vi "Launch XY Config Dialog.vi"(8 "error in (no error)":errorcluster, 11 "Waveform Graph Data in":T1={"Custom Data"=variant, "EventRegs"={"SystemChange"=refnum, "WorkspaceState"=refnum, "Graph"=refnum, "Wks&Dialog&Periodic"=refnum}, "References"={"X.Scale.Auto"=refnum, "Y.Scale.Auto"=refnum, "X.Scale.Once"=refnum, "Y.Scale.Once"=refnum, "LegendVis"=refnum, "Graph"=refnum}, "Persistent Data"={"Label"="", "Graph Props"={"Plots"=[], "Legend:Number of Rows"=0, "Scale Properties"={"X.Auto"=FALSE, "X.Min"=0.0, "X.Max"=0.0, "X.IgnoreTS"=FALSE, "X.Precision"=0, "X.Label:"="", "X.LabelVis"=FALSE, "X.DefLabel"=FALSE, "Y.Auto"=FALSE, "Y.Min"=0.0, "Y.Max"=0.0, "Y.Format"=0, "Y.Precision:"=0, "Y.Label:"="", "Y.LabelVis"=FALSE, "Y.DefLabel"=FALSE, "X.Format"=0}, "Legend:Visible"=TRUE, "BgColor"=0, "Last Plot Width"=0, "Resize"=FALSE}, "UDP Data"={"Decimation"=0, "UDP Buffer Size"=0, "History Length"=0.0, "Update Rate"=enum."15 Hz", "Channel Paths"=[], "Channel Names"=[]}}, "System"={"To Workspace"=refnum, "From Workspace"=refnum, "NIVS helper"=refnum, "Gtwy"="", "Root"=refnum, "Workspace"=refnum, "SystemStateRefs"={"CustDatRef"=refnum, "EvtRef"=refnum}, "Connected?"=FALSE, "FromDialog"=refnum, "ErrFlag"=FALSE, "New"=FALSE, "ErrState"="", "Save"=FALSE, "Hold"=FALSE, "Periodic"=refnum, "ToDialog"=refnum, "DialogEventReg"=refnum, "UseSavedWidth"=FALSE, "TreeBrowserEventReg"=refnum, "UDPChannelStreamSession"=refnum, "Valid Channels?"=FALSE, "Update Graph"=refnum, "UDP Queue"=refnum, "Graph Update Queue"=refnum}, "GraphData"=[], "UDP Stream Active?"=FALSE} {"Persistent Data"."Graph Props"."Scale Properties"."X.Format" items=["Decimal", "Scientific", "Engineering", "Binary", "Octal", "Hexadecimal", "Relative Time", "Time and Date", "SI", "Automatic"]; "Persistent Data"."Graph Props"."Scale Properties"."Y.Precision:" items=["0", "1", "2", "3", "4", "5", "6", "7"]; "Persistent Data"."Graph Props"."Scale Properties"."Y.Format" items=["Decimal", "Scientific", "Engineering", "Binary", "Octal", "Hexadecimal", "Relative Time", "Time and Date", "SI", "Automatic"]; "Persistent Data"."Graph Props"."Scale Properties"."X.Precision" items=["0", "1", "2", "3", "4", "5", "6", "7"]}) -> (0 "error out":errorcluster)   [LabVIEW 2013, in "Workspace MultiY Graph.lvlib"]
uses:
  Workspace MultiY Graph.lvlib
  XY Top level workspace graph data.ctl
  <vilib>/NI Veristand/Execution/Workspace/SystemStateRegEventRef.ctl
  <vilib>/NI Veristand/Display Template Support/Display Template Support.llb/enum_Display Template Handler Minimal To Widget Msg.ctl
  XY Dialog Msg to Control.ctl
  XY Dialog Msg Type.ctl
  XY Persistent Data.ctl
  XY Graph Properties.ctl
  XY Plot Properties.ctl
  XY Scale Properties.ctl
  XY Scale Precision.ctl
  XY Scale Format.ctl
  UDP Data.ctl
  Update Rate.ctl
  XY References.ctl
  <vilib>/NI Veristand/Display Template Support/Display Template Support.llb/enum_Display Template Handler Minimal To Workspace.ctl
  NationalInstruments.VeriStand.SystemStorage
  <vilib>/NI Veristand/Execution/Workspace/WorkspaceAPI.ctl
  NationalInstruments.VeriStand.ClientAPI
  <vilib>/NI Veristand/Execution/Workspace/SystemStateEventRef.ctl
  XY Control Msg to Dialog.ctl
  <vilib>/NI Veristand/UI Controls/Tree and Alias Browser/Net Event Data Ref.ctl
  <vilib>/NI Veristand/UI Controls/Tree and Alias Browser/Net Event Data.ctl
  <vilib>/NI Veristand/UI Controls/Tree and Alias Browser/Net Event.ctl
  <vilib>/NI Veristand/Execution/Workspace/UDPChannelStreamSession.ctl
  UDP Queue Data.ctl
  UDP Action State.ctl
  Graph Update Queue Data.ctl
  Graph Update Action State.ctl
  Dlg Symbol.ctl
  Alert Dialogs.lvlib
  <vilib>/NI Veristand/Execution/Workspace/NI_VS Workspace ExecutionAPI.lvlib
  <vilib>/NI Veristand/UI Controls/Tree and Alias Browser/NI_VS UI Tree Alias Browser.lvlib
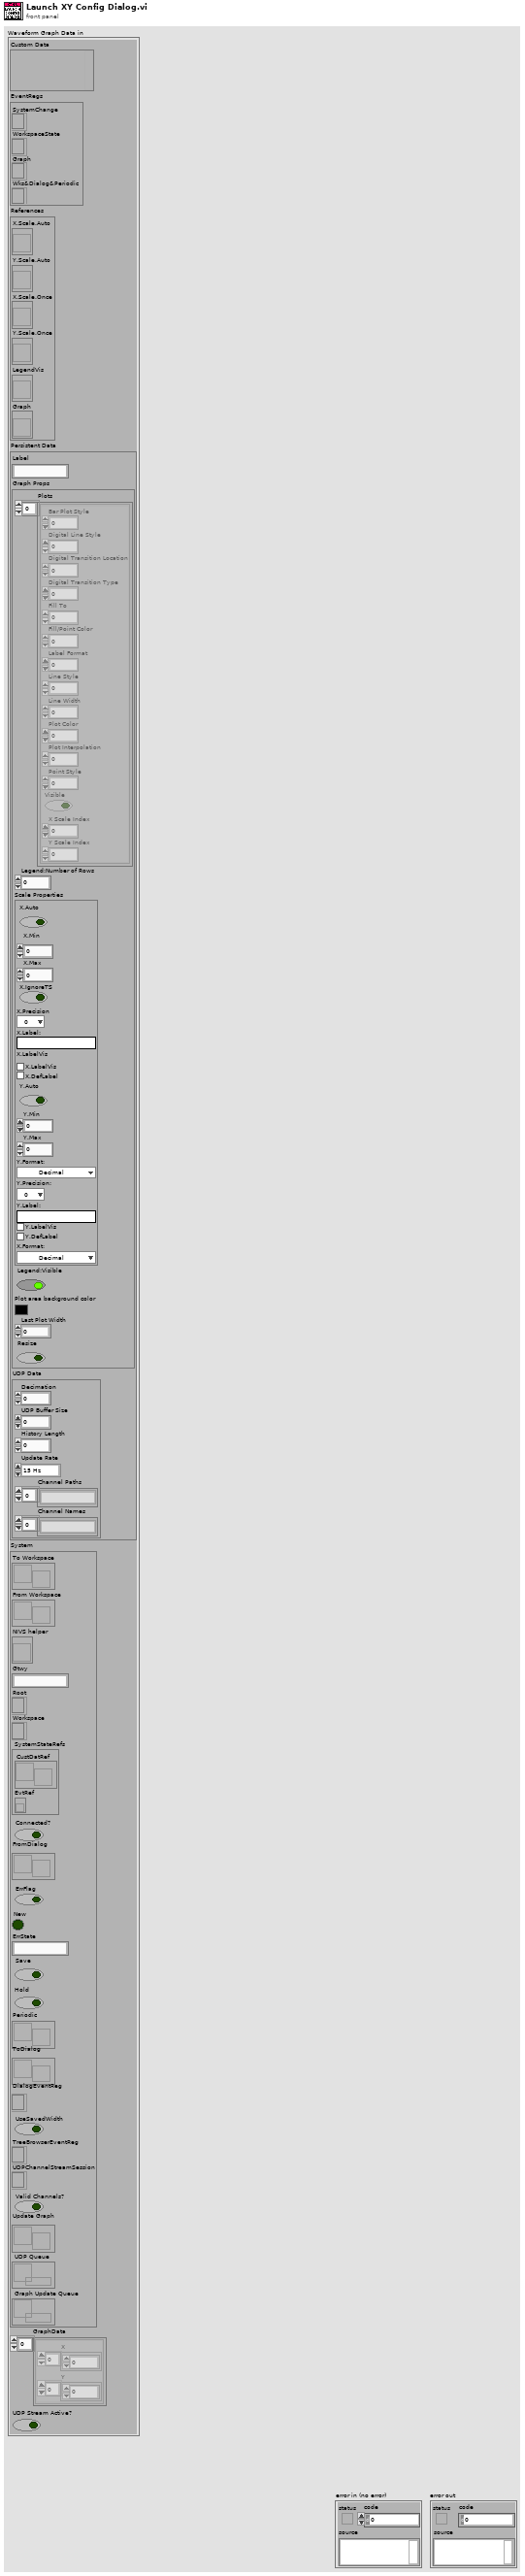
[diagram p1: front panel]
types:
  T1 = typedef "Workspace MultiY Graph.lvlib/XY Top level workspace graph data.ctl" = cluster{"Custom Data":variant, "EventRegs":cluster{"SystemChange":T2, "WorkspaceState":refnum<event-registration>, "Graph":refnum<event-registration>, "Wks&Dialog&Periodic":refnum<event-registration>}, "References":T3, "Persistent Data":T4, "System":cluster{"To Workspace":refnum<user-event>, "From Workspace":refnum<user-event>, "NIVS helper":refnum<vi>, "Gtwy":string, "Root":refnum<k24>, "Workspace":T12, "SystemStateRefs":T13, "Connected?":bool, "FromDialog":refnum<user-event>, "ErrFlag":bool, "New":bool, "ErrState":string, "Save":bool, "Hold":bool, "Periodic":refnum<user-event>, "ToDialog":refnum<user-event>, "DialogEventReg":refnum<event-registration>, "UseSavedWidth":bool, "TreeBrowserEventReg":refnum<event-registration>, "UDPChannelStreamSession":T14, "Valid Channels?":bool, "Update Graph":refnum<user-event>, "UDP Queue":refnum<queue>, "Graph Update Queue":refnum<queue>}, "GraphData":cluster{"X":dbl[], "Y":dbl[]}[], "UDP Stream Active?":bool}
  T2 = typedef "NI_VS Workspace ExecutionAPI.lvlib/SystemStateRegEventRef.ctl" = refnum<event-registration>
  T3 = typedef "Workspace MultiY Graph.lvlib/XY References.ctl" = cluster{"X.Scale.Auto":refnum<vi>, "Y.Scale.Auto":refnum<vi>, "X.Scale.Once":refnum<vi>, "Y.Scale.Once":refnum<vi>, "LegendVis":refnum<vi>, "Graph":refnum<vi>}
  T4 = typedef "Workspace MultiY Graph.lvlib/XY Persistent Data.ctl" = cluster{"Label":string, "Graph Props":T5, "UDP Data":T10}
  T5 = typedef "Workspace MultiY Graph.lvlib/XY Graph Properties.ctl" = cluster{"Plots":T6[], "Legend:Number of Rows":u32, "Scale Properties":T7, "Legend:Visible":bool, "BgColor":u32, "Last Plot Width":u32, "Resize":bool}
  T6 = typedef "Workspace MultiY Graph.lvlib/XY Plot Properties.ctl" = cluster{"Bar Plot Style":u8, "Digital Line Style":u8, "Digital Transition Location":u8, "Digital Transition Type":u8, "Fill To":i16, "Fill/Point Color":u32, "Label Format":u8, "Line Style":u8, "Line Width":u8, "Plot Color":u32, "Plot Interpolation":u8, "Point Style":u8, "Visible":bool, "X Scale Index":u32, "Y Scale Index":u32}
  T7 = typedef "Workspace MultiY Graph.lvlib/XY Scale Properties.ctl" = cluster{"X.Auto":bool, "X.Min":dbl, "X.Max":dbl, "X.IgnoreTS":bool, "X.Precision":T8, "X.Label:":string, "X.LabelVis":bool, "X.DefLabel":bool, "Y.Auto":bool, "Y.Min":dbl, "Y.Max":dbl, "Y.Format":T9, "Y.Precision:":T8, "Y.Label:":string, "Y.LabelVis":bool, "Y.DefLabel":bool, "X.Format":T9}
  T8 = typedef "Workspace MultiY Graph.lvlib/XY Scale Precision.ctl" = u8
  T9 = typedef "Workspace MultiY Graph.lvlib/XY Scale Format.ctl" = u8
  T10 = typedef "Workspace MultiY Graph.lvlib/UDP Data.ctl" = cluster{"Decimation":i32, "UDP Buffer Size":u32, "History Length":dbl, "Update Rate":T11, "Channel Paths":string[], "Channel Names":string[]}
  T11 = typedef "Workspace MultiY Graph.lvlib/Update Rate.ctl" = enum8{"15 Hz", "10 Hz", "5 Hz", "4 Hz", "3 Hz", "2 Hz", "1 Hz", "0.5 Hz"}
  T12 = typedef "NI_VS Workspace ExecutionAPI.lvlib/WorkspaceAPI.ctl" = refnum<k24>
  T13 = typedef "NI_VS Workspace ExecutionAPI.lvlib/SystemStateEventRef.ctl" = cluster{"CustDatRef":refnum<user-event>, "EvtRef":refnum<k27>}
  T14 = typedef "NI_VS Workspace ExecutionAPI.lvlib/UDPChannelStreamSession.ctl" = refnum<k24>
  T15 = enum16{"Default", "Administration", "Channel Scaling Utility", "Add Display Items", "Change User Profile", "Edit Stimulus Profile Editor Header", "Edit Display Item Settings", "Model Parameter Calibration", "Runtime Alarm Edit", "Edit Tools Menu", "Edit Engine Components", "Configure Visible Channels", "Fault Manager"}
  T16 = typedef "Workspace MultiY Graph.lvlib/Alert Dialogs.lvlib/Dlg Symbol.ctl" = enum16{"Information", "Help", "Warning", "Error"}
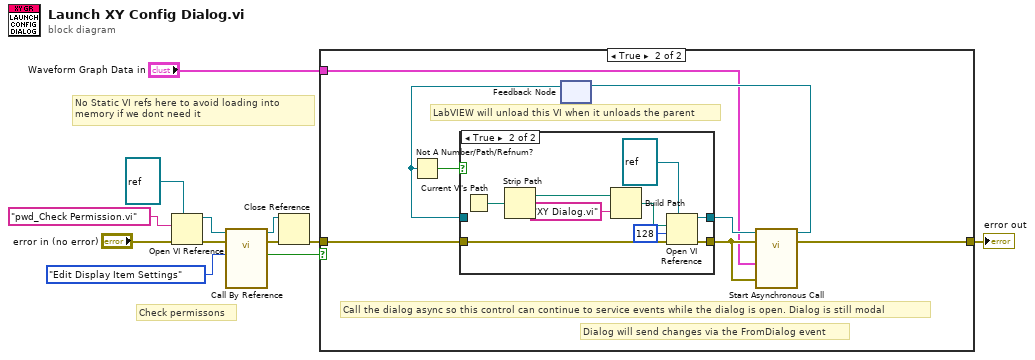
[diagram p0: block diagram]
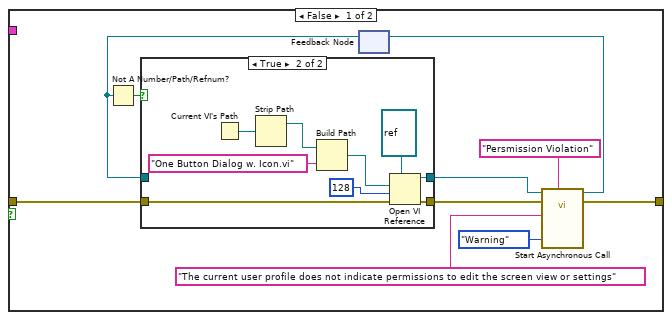
[diagram p2: hidden frame]
diagram:
  # "No Static VI refs here to avoid loading into memory if we dont need it"
  # "Check permissons"
  n1 = Open VI Reference(type specifier VI Refnum (for type only)=refnum<vi> refnum, vi path="pwd_Check Permission.vi", error in (no error)="error in (no error)") -> (vi reference=w8:refnum<vi>, error out=w9:errorcluster)  [unwired: 3 in]
  n2 = call-by-ref "?"(reference=w8, error in=w9, "Permission"=T15."Edit Display Item Settings") -> (reference out=w4:refnum<vi>, error out=w6:errorcluster, "Valid"=w3:bool)  [unwired: 18 in]
  n3 = Close Reference(reference=w4, error in (no error)=w6) -> (error out=w5:errorcluster)
  n4 = case shown="True" w3 {
    tunnel: [w16 w39] -> w2
    tunnel: w5 -> [w20 w40]
    tunnel: "Waveform Graph Data in" -> [_ w34]
    frame False {
      n5 = feedback #1() -> (w13:refnum<vi>)  [unwired: 1 in]
      n6 = Not A Number/Path/Refnum?(number/path/refnum=w13) -> (NaN/Path/Refnum?=w15:bool)
      n7 = case shown="True" w15 {
        tunnel: [w24 w33] -> w22
        tunnel: [w23 w32] -> w21
        tunnel: w20 -> [w23 w31]
        tunnel: w13 -> [w24 _]
        frame False {
        }
        frame True {
          n8 = Current VI's Path() -> (path=w26:path)
          n9 = Strip Path(path=w26) -> (stripped path=w25:path)  [unwired: 1 out]
          n10 = Build Path(base path=w25, name or relative path="One Button Dialog w. Icon.vi") -> (appended path=w28:path)
          n11 = Open VI Reference(type specifier VI Refnum (for type only)=refnum<vi> refnum, vi path=w28, options=128, error in (no error)=w31) -> (vi reference=w33:refnum<vi>, error out=w32:errorcluster)  [unwired: 2 in]
        }
      }
      n12 = call-by-ref "Start Asynchronous Call"(reference=w22, error in=w21, "Window Title (\"\")"="Persmission Violation" ("Window Title (\"\")"), "Symbol"=Dlg_Symbol."Warning", "message"="The current user profile does not indicate permissions to edit the screen view or settings") -> (reference out=w14:refnum<vi>, error out=w16:errorcluster)  [unwired: 8 in, 1 out]
      n13 = feedback-in #1(w14) -> ()
    }
    frame True {
      # "LabVIEW will unload this VI when it unloads the parent"
      # "Dialog will send changes via the FromDialog event"
      # "Call the dialog async so this control can continue to service events while the dialog is open. Dialog is still modal"
      n14 = feedback #2() -> (w36:refnum<vi>)  [unwired: 1 in]
      n15 = Not A Number/Path/Refnum?(number/path/refnum=w36) -> (NaN/Path/Refnum?=w38:bool)
      n16 = case shown="True" w38 {
        tunnel: [w43 w52] -> w35
        tunnel: [w42 w51] -> w41
        tunnel: w40 -> [w43 w50]
        tunnel: w36 -> [w42 _]
        frame False {
        }
        frame True {
          n17 = Current VI's Path() -> (path=w46:path)
          n18 = Strip Path(path=w46) -> (stripped path=w45:path)  [unwired: 1 out]
          n19 = Build Path(base path=w45, name or relative path="XY Dialog.vi") -> (appended path=w47:path)
          n20 = Open VI Reference(type specifier VI Refnum (for type only)=refnum<vi> refnum, vi path=w47, options=128, error in (no error)=w50) -> (vi reference=w51:refnum<vi>, error out=w52:errorcluster)  [unwired: 2 in]
        }
      }
      n21 = call-by-ref "Start Asynchronous Call"(reference=w41, error in=w35, 8:"error in (no error)"=w35, "Waveform Graph Data in"=w34) -> (reference out=w37:refnum<vi>, error out=w39:errorcluster)  [unwired: 10 in]
      n22 = feedback-in #2(w37) -> ()
    }
  }
  "error out" <- w2
